vi "efficiency_test.vi"() -> ()   [LabVIEW 2020, in "efficiency_test.lvlib"]
uses:
  efficiency_test.lvlib
  typedefs/test_inputs.ctl
  typedefs/test_results.ctl
  typedefs/instrument_resources.ctl
  <vilib>/addons/_JKI Toolkits/State Machine/_JKI_lib_State_Machine.llb/Select State(s)_err__jki_lib_state_machine.vi
  drivers/Agilent 34401/Public/Data/Read (Single Point).vi
  drivers/Agilent 34401/Agilent 34401.lvlib
  drivers/Agilent 33XXX Series/Agilent 33XXX Series.lvlib
  drivers/Agilent E364X Series/Agilent E364X Series.lvlib
  drivers/Agilent B2900 Series/Agilent B2900 Series.lvlib
panel:
  in  "UI Tab":enum32{"Test", "Instrument Resources"}(tab)
  out "Efficiency (%) vs ILoad (A)":T1(graph) caption="XY Graph - dark"
  in  "test_inputs":T2={"Vin (V)"=36.0, "Iin Limit (A)"=0.1, "ILoad Start (A)"=0.0, "ILoad Stop (A)"=10.0, "ILoad Step (A)"=1.0, "Vdd (V)"=36.0, "IVdd Limit (A)"=0.1} {"IVdd Limit (A)" format="%#_6p"; "Vdd (V)" format="%#_6p"; "ILoad Step (A)" format="%#_6p"; "ILoad Stop (A)" format="%#_6p"; "ILoad Start (A)" format="%#_6p"; "Iin Limit (A)" format="%#_6p"; "Vin (V)" format="%#_6p"}
  out "Output Results":T3
  in  "instrument_resources":T4={"Vin Voltage DMM"="Vin_Volt", "Vin Current DMM"="Vin_Current", "Vout Voltage DMM"="Vout Voltage DMM", "Vout Current DMM"="Vout_Current", "Eload"="Eload", "FSW_Source"="FSW", "Vin_supply"="Vin_supply", "Vdd_supply"="Vin_supply"}
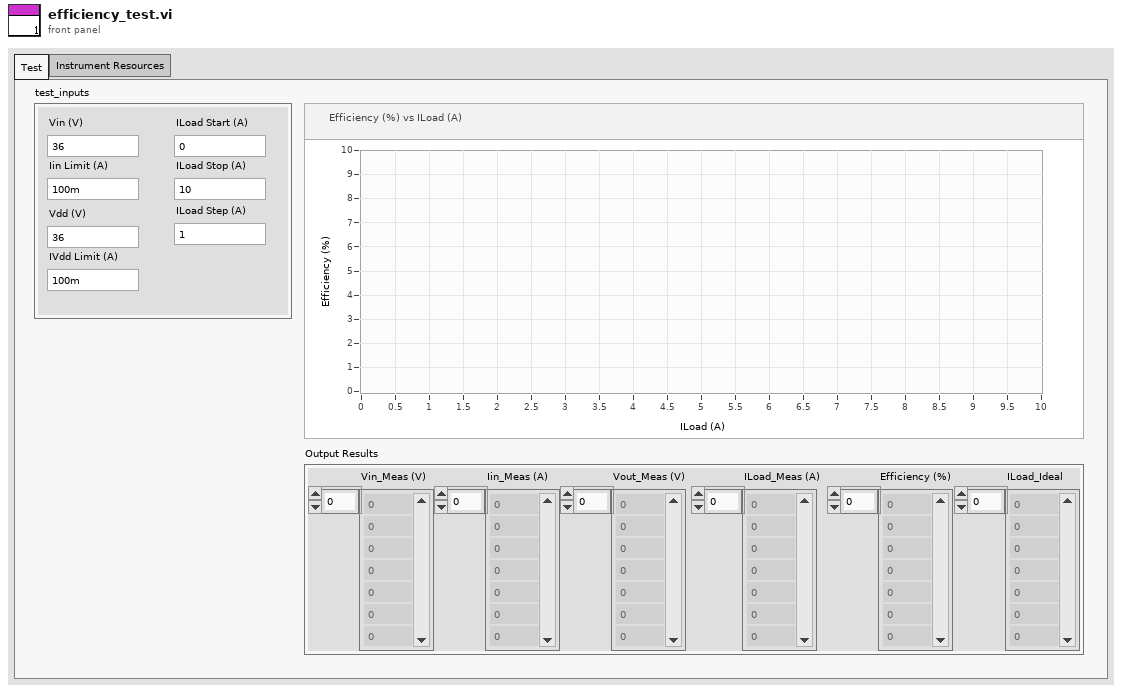
[diagram p1: front panel]
types:
  T1 = cluster{"ILoad (A)":dbl[], "Efficiency (%) ":dbl[]}
  T2 = typedef "efficiency_test.lvlib/test_inputs.ctl" = cluster{"Vin (V)":dbl, "Iin Limit (A)":dbl, "ILoad Start (A)":dbl, "ILoad Stop (A)":dbl, "ILoad Step (A)":dbl, "Vdd (V)":dbl, "IVdd Limit (A)":dbl}
  T3 = typedef "efficiency_test.lvlib/test_results.ctl" = cluster{"Vin_Meas (V)":dbl[], "Iin_Meas (A)":dbl[], "Vout_Meas (V)":dbl[], "ILoad_Meas (A)":dbl[], "Efficiency (%)":dbl[], "ILoad_Ideal":dbl[]}
  T4 = typedef "efficiency_test.lvlib/instrument_resources.ctl" = cluster{"Vin Voltage DMM":refnum<visa-resource-name>, "Vin Current DMM":refnum<visa-resource-name>, "Vout Voltage DMM":refnum<visa-resource-name>, "Vout Current DMM":refnum<visa-resource-name>, "Eload":refnum<visa-resource-name>, "FSW_Source":refnum<visa-resource-name>, "Vin_supply":refnum<visa-resource-name>, "Vdd_supply":refnum<visa-resource-name>}
  T5 = cluster{"test_inputs":T2, "output_results":T3, "instrument_resources":T4, "ILoad Sweep Current":dbl[]}
  T6 = cluster{"ILoad_Meas (A)":dbl[], "Efficiency (%)":dbl[]}
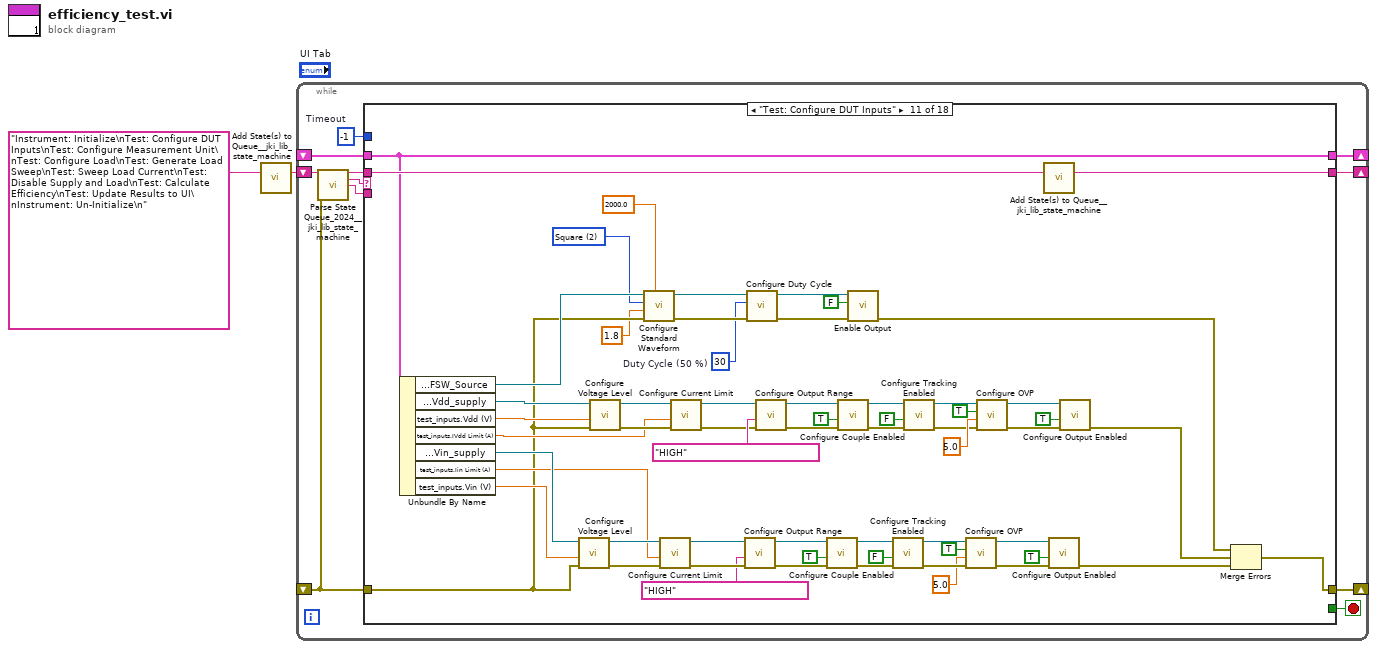
[diagram p0: block diagram]
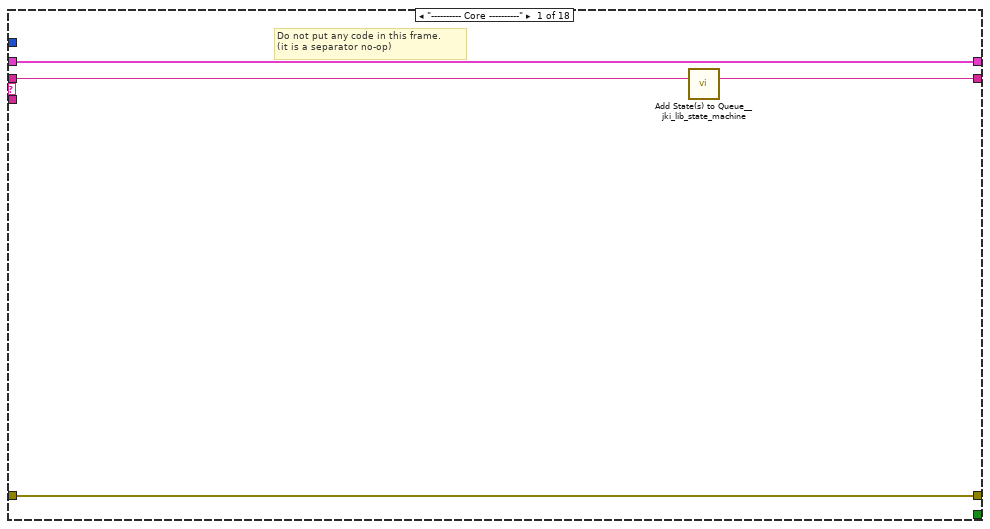
[diagram p2: hidden frame]
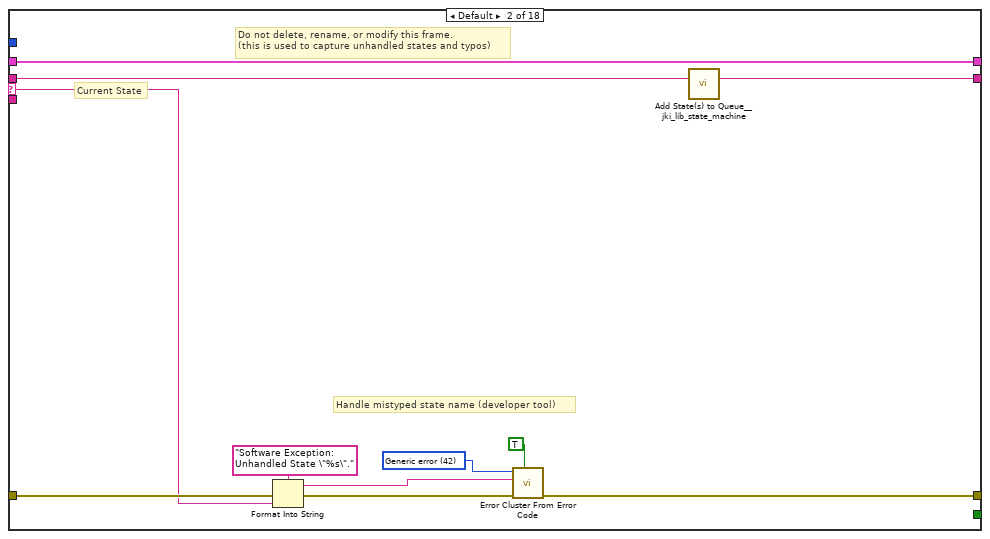
[diagram p3: hidden frame]
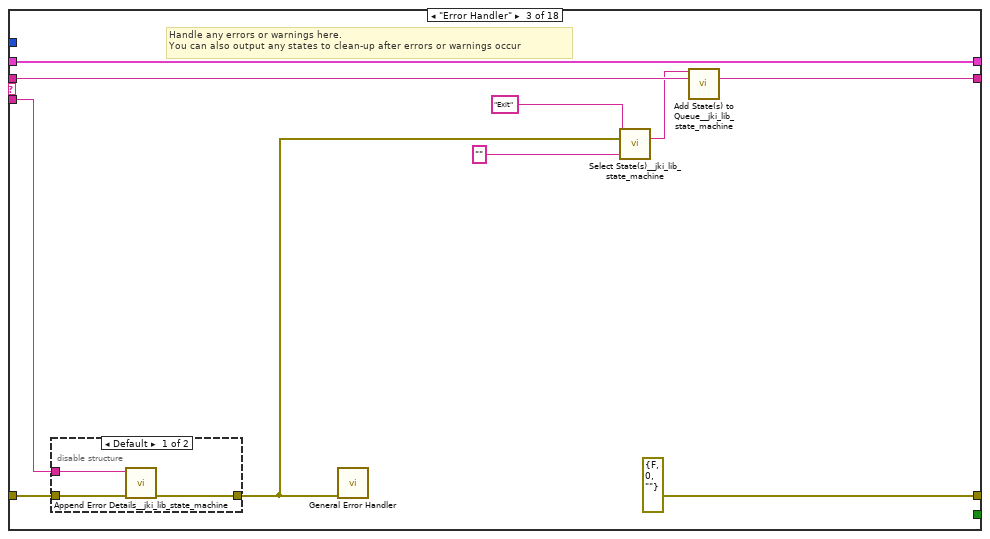
[diagram p4: hidden frame]
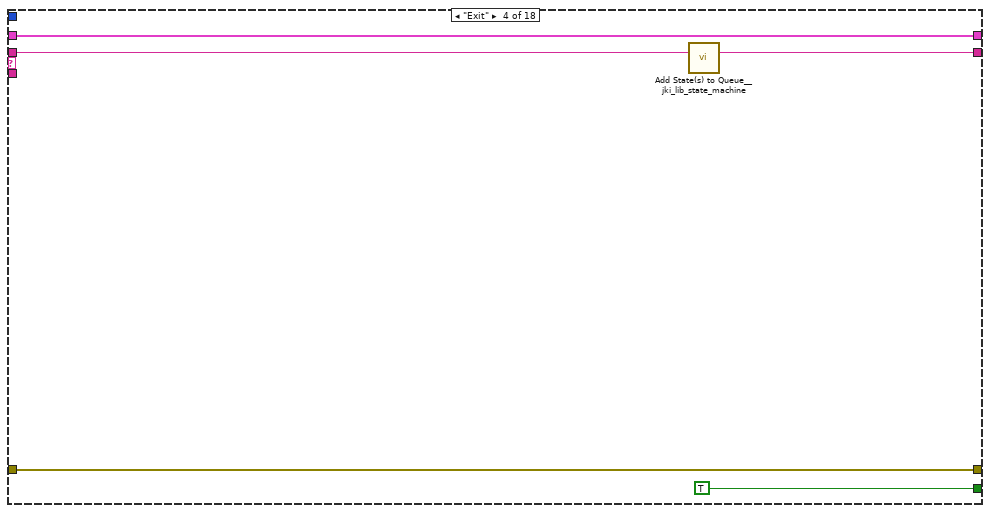
[diagram p6: hidden frame]
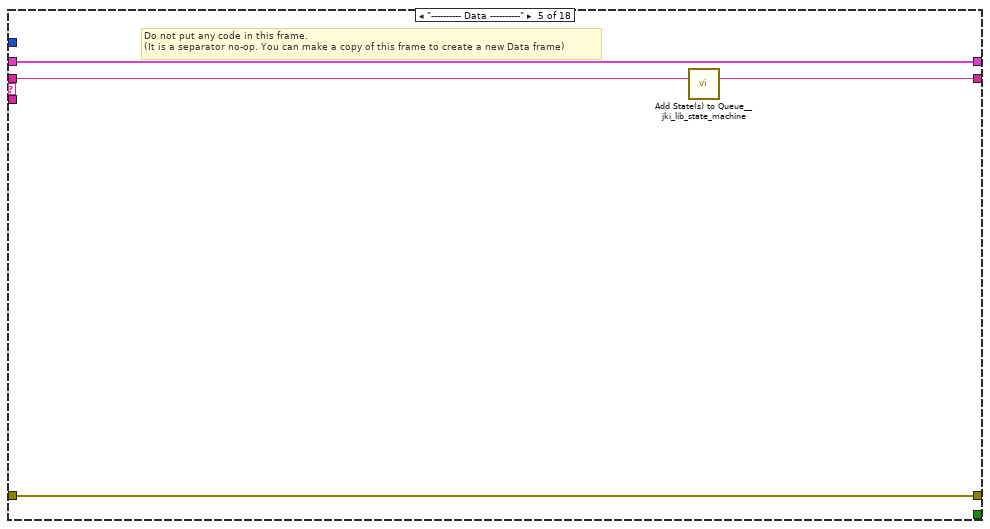
[diagram p7: hidden frame]
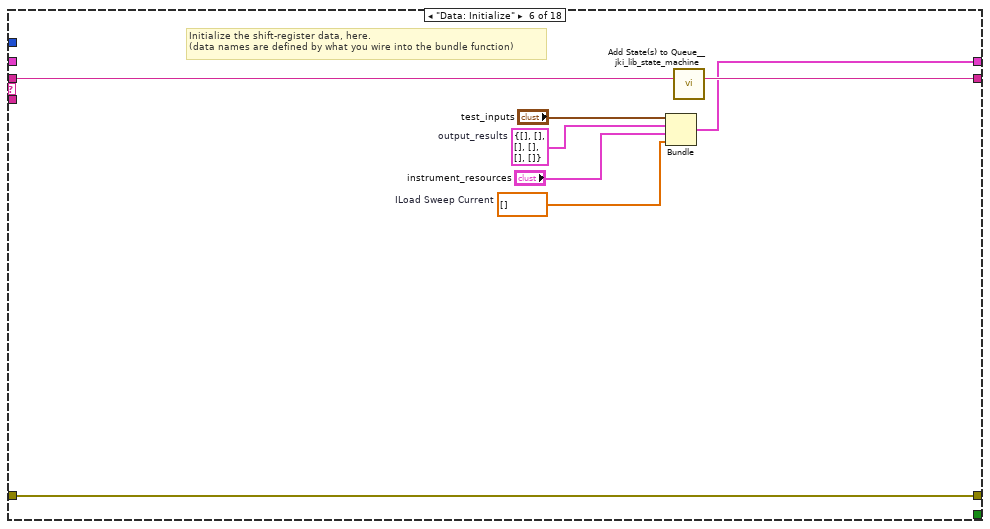
[diagram p8: hidden frame]
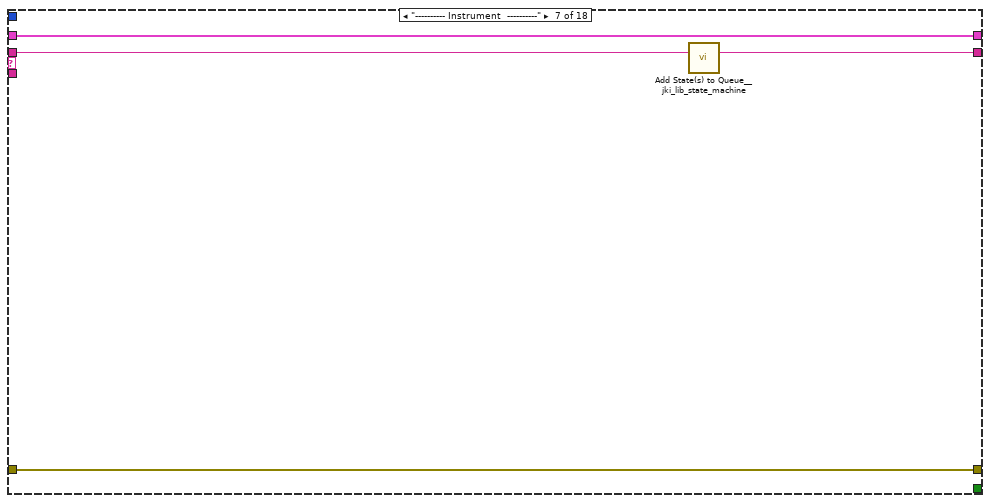
[diagram p9: hidden frame]
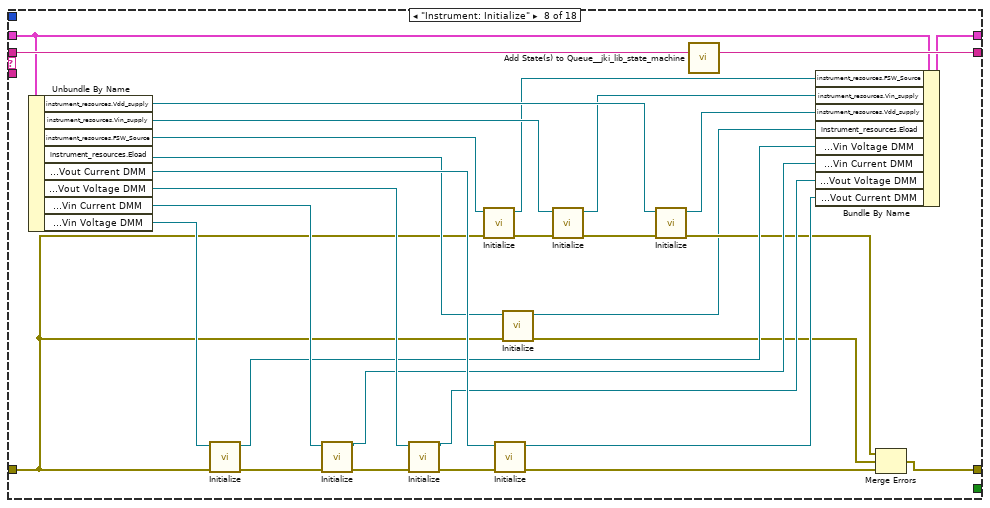
[diagram p10: hidden frame]
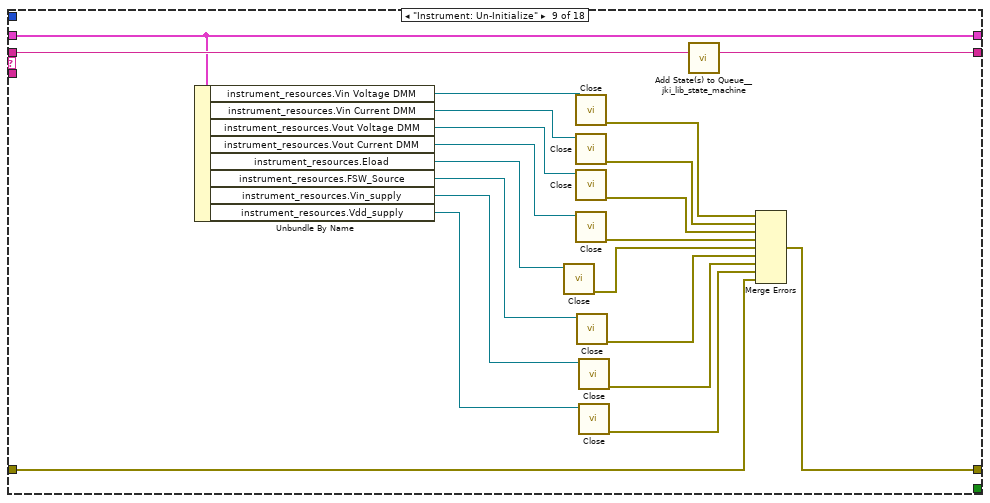
[diagram p11: hidden frame]
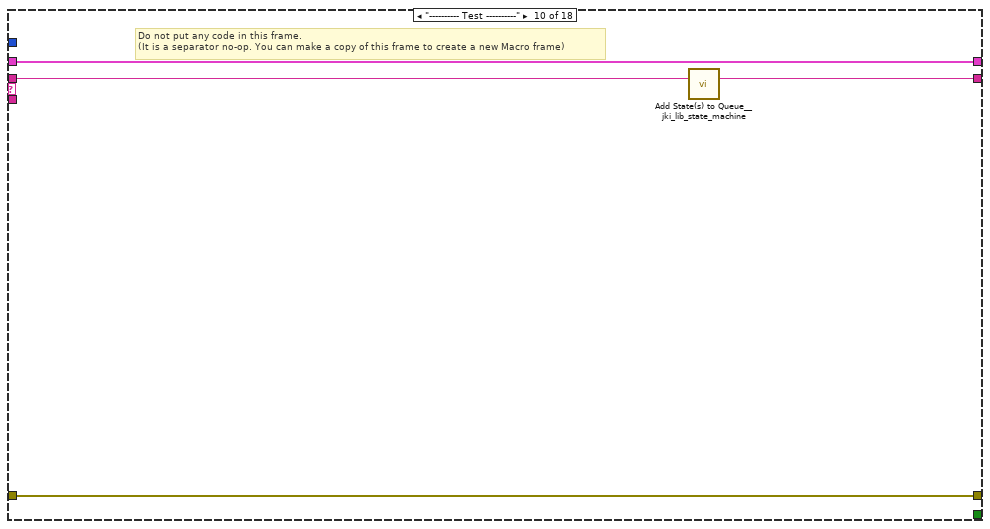
[diagram p12: hidden frame]
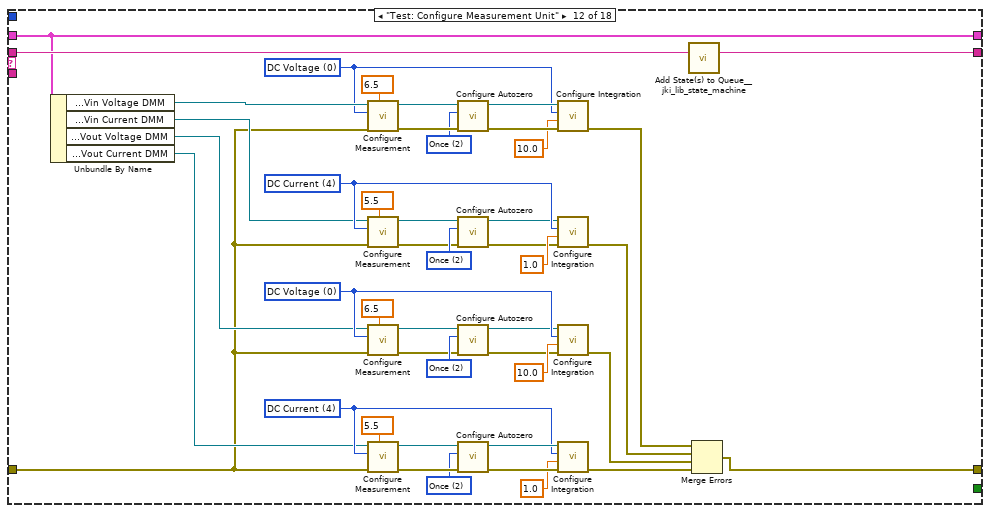
[diagram p13: hidden frame]
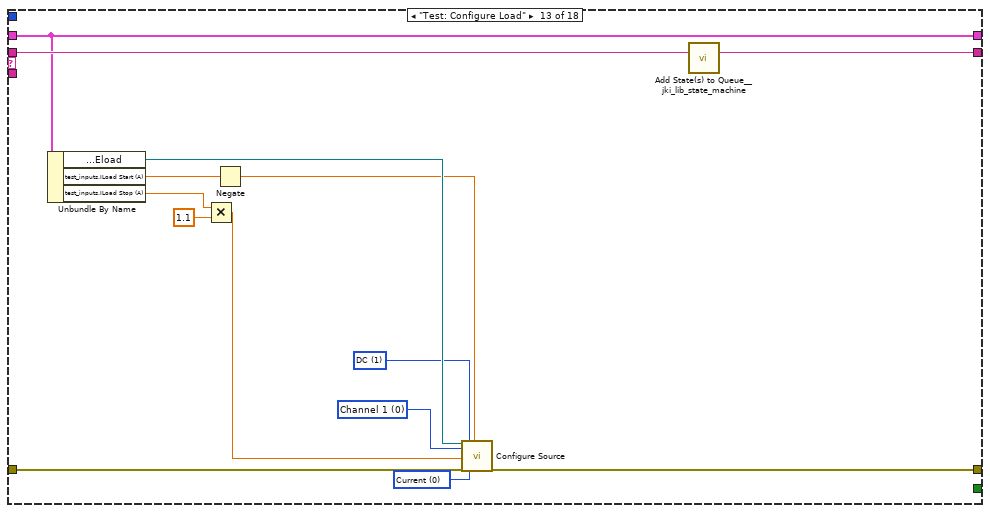
[diagram p14: hidden frame]
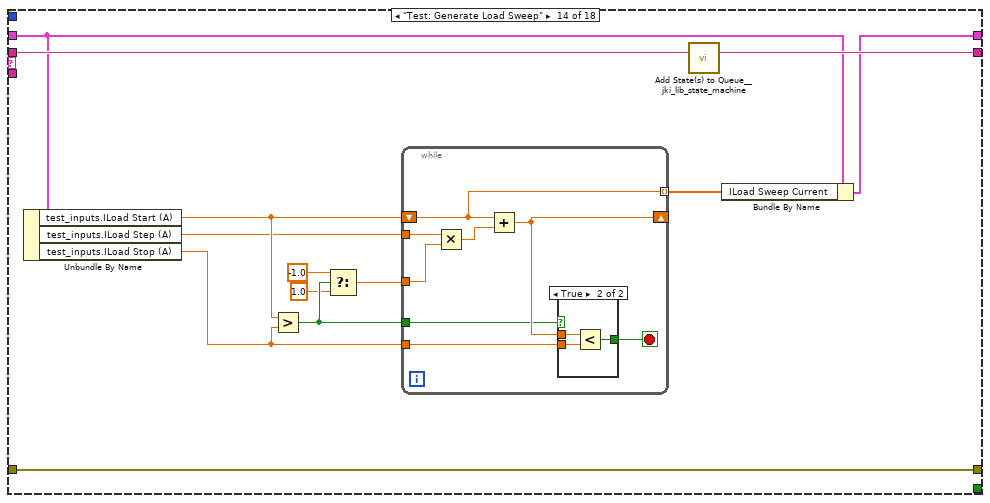
[diagram p15: hidden frame]
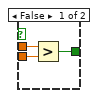
[diagram p16: hidden frame]
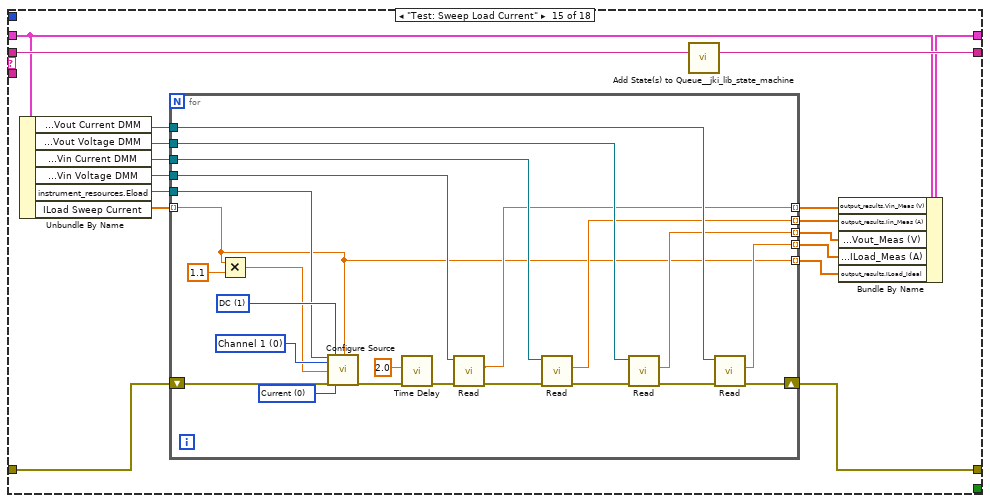
[diagram p17: hidden frame]
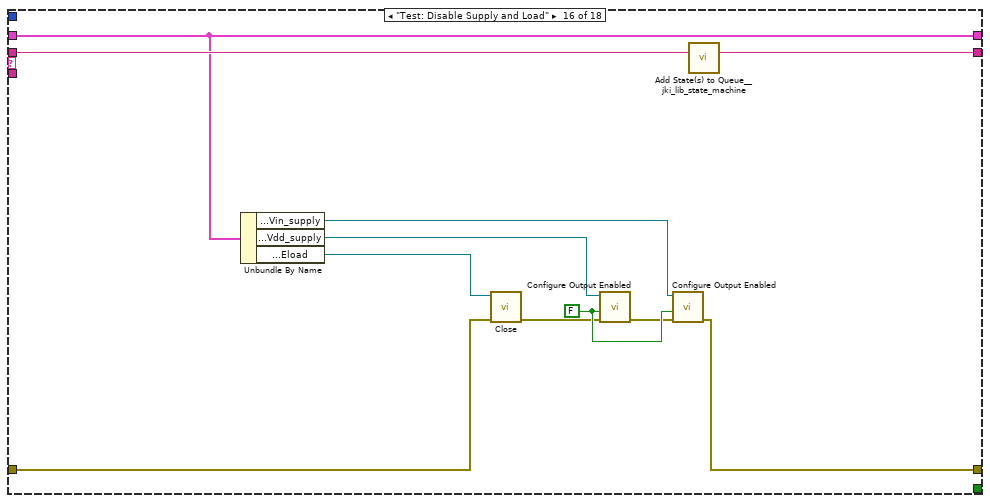
[diagram p18: hidden frame]
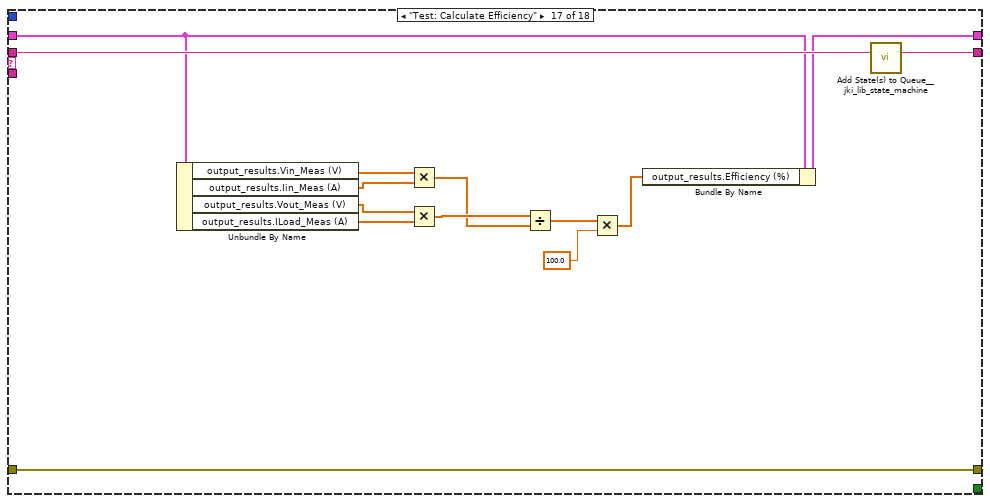
[diagram p19: hidden frame]
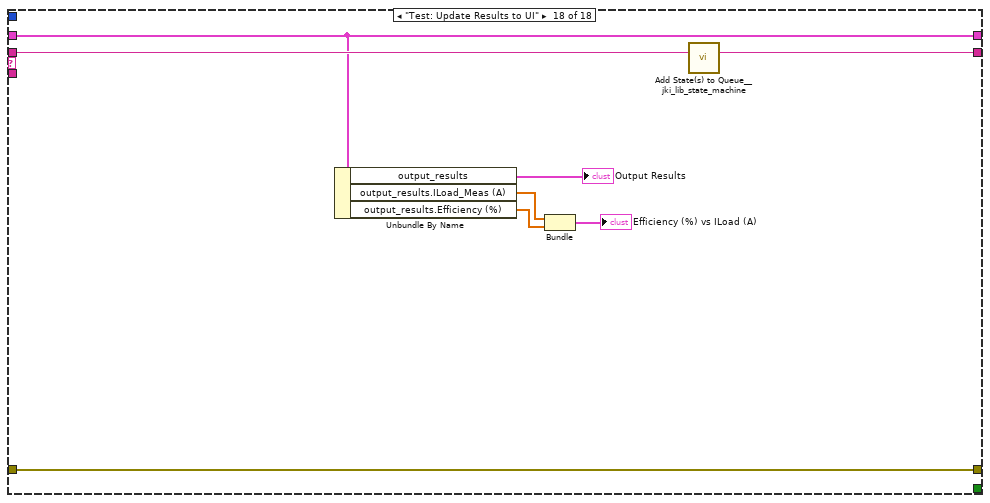
[diagram p20: hidden frame]
diagram:
  n1 = call <vilib>:"Add State(s) to Queue__jki_lib_state_machine.vi"("State(s) in (\"\")"="Instrument: Initialize\nTest: Configure DUT Inputs\nTest: Configure Measurement Unit\nTest: Configure Load\nTest: Generate Load Sweep\nTest: Sweep Load Current\nTest: Disable Supply and Load\nTest: Calculate Efficiency\nTest: Update Results to UI\nInstrument: Un-Initialize\n") -> ("States Out"=w2:string)  [unwired: 14 in]
  n2 = while {
    shift-right: [w6] -> _
    shift-left: _ -> [w5]
    shift-right: [w9] -> _
    shift-left: _ -> [w3]
    shift-right: [w8] -> _
    shift-left: w2 -> [w10]
    stop <- w7 stop-if-true
    w4 = -1  # Timeout
    n3 = call <vilib>:"Parse State Queue_2024__jki_lib_state_machine.vi"("State Queue"=w10, "Error In (no error)"=w3) -> ("Remaining States"=w12:string, "Current State"=w13:string, "Arguments"=w11:string)  [unwired: 11 in]
    n4 = case shown="\"Test: Configure DUT Inputs\"" w13 {
      selector: w13 -> [_ w18 _ _ _ _ _ _ _ _ _ _ _ _ _ _ _ _]
      tunnel: w12 -> [w17 w22 w38 w47 w51 w59 w63 w93 w114 w118 w178 w223 w237 w250 w281 w315 w329 w337]
      tunnel: w11 -> [_ _ w33 _ _ _ _ _ _ _ _ _ _ _ _ _ _ _]
      tunnel: w5 -> [w14 w20 w35 w45 w48 _ w60 w71 w112 w115 w176 w221 w235 w238 w267 w313 w316 w334]
      tunnel: [w15 w24 errorcluster {"status"=FALSE, "code"=0, "source"=""} ("error out") w44 w49 w56 w61 w68 w97 w116 w119 w179 w230 w248 w266 w308 w327 w335] -> w9
      tunnel: w3 -> [w15 w23 w34 w44 w49 w56 w61 w65 w96 w116 w132 w184 w231 w248 w265 w306 w327 w335]
      tunnel: [w16 w21 w37 w46 w50 w58 w62 w92 w113 w117 w177 w222 w236 w249 w280 w314 w328 w336] -> w8
      tunnel: [_ _ _ TRUE _ _ _ _ _ _ _ _ _ _ _ _ _ _] -> w7
      tunnel: [w14 w20 w35 w45 w48 w57 w60 w72 w112 w115 w176 w221 w235 w239 w268 w313 w317 w334] -> w6
      tunnel: w4 -> [_ _ _ _ _ _ _ _ _ _ _ _ _ _ _ _ _ _]
      frame "---------- Core ----------" {
        # "Do not put any code in this frame.\n(it is a separator no-op)"
        n5 = call <vilib>:"Add State(s) to Queue__jki_lib_state_machine.vi"("State(s) in (\"\")"=w17) -> ("States Out"=w16:string)  [unwired: 14 in]
      }
      frame Default {
        w27 = 42 items=["No error", "Argument error", "Memory is full", "Out of zone", "End of file", "File already open", "Generic file I/O error", "File not found", "File permission error", "Disk is full", "Duplicate path", "Too many files open", "System feature not enabled", "Resource file not found", "Cannot add resource", "Resource not found", "Image not found", "Image memory error", "Pen does not exist", "Config type invalid", "Config token not found", "Config parse error", "Config memory error", "Bad external code format", "Bad external code offset", "External code not present", "Null window", "Destroy window error", "Null menu", "Print aborted", "Bad print record", "Print driver error", "Windows error during printing", "Memory error during printing", "Print dialog error", "Generic print error", "Invalid device refnum", "Device not found", "Device parameter error", "Device unit error", "Cannot open device", "Device call aborted", "Generic error", "Cancelled by user", "Object ID too low", "Object ID too high", "Object not in heap", "Unknown heap", "Unknown object (invalid DefProc)", "Unknown object (DefProc not in table)", "Message out of range", "Invalid (null) method", "Unknown message", "Manager call not supported", "Bad address", "Network operation in progress", "Network operation timed out", "Connection is busy", "Network attribute not supported", "Network error", "Address in use", "System out of memory", "Connection aborted", "Connection refused", "Not connected", "Already connected", "Connection closed", "Initialization error (interapplication manager)", "Bad occurrence", "Wait on unbound occurrence handler", "Occurrence queue overflow", "Datalog type conflict", "Unused", "Unrecognized type (interapplication manager)", "Memory corrupt", "Failed to make temporary DLL", "Old CIN version", "Drag socket not found", "Failed to load drop-object", "Failed to register OLE object", "Failed to release OLE object", "Format specifier type mismatch", "Unknown format specifier", "Too few format specifiers", "Too many format specifiers", "Scan failed", "Newer CIN version", "Error converting to variant", "Runtime menu error", "Password tampered", "Variant attribute not found", "Incompatible variant data type", "Event data is not available", "Event Store is not present", "Occurrence is not found", "Event Queue is not created", "Event info is not available", "Refnum passed is NULL", "Error retrieving Class GUID", "Error retrieving CoClass GUID", "Error retrieving TypeLib GUID.", "Bad built application magic bytes.", "Specific driver is different from the specific driver associated with the Logical Name.", "There is no session opened to the class driver.", "Max Error", "MAX - Error with config objects", "MAX - Error loading configuration", "MAX - Group not supported"]
        # "Current State"
        # "Do not delete, rename, or modify this frame.\n(this is used to capture unhandled states and typos)"
        # "Handle mistyped state name (developer tool)"
        n6 = Format Into String(format string="Software Exception: Unhandled State \"%s\"." ("message"), error in=w23, w18) -> (resulting string=w26:string, error out=w25:errorcluster)  [unwired: 1 in]
        n7 = call <vilib>:"Error Cluster From Error Code.vi"("show call chain? (False)"=TRUE, "error in (no error)"=w25, "error message (\"\")"=w26, "error code (0)"=w27) -> ("error out"=w24:errorcluster)  [unwired: 5 in]
        n8 = call <vilib>:"Add State(s) to Queue__jki_lib_state_machine.vi"("State(s) in (\"\")"=w22) -> ("States Out"=w21:string)  [unwired: 14 in]
      }
      frame "Error Handler" {
        # "Handle any errors or warnings here.\nYou can also output any states to clean-up after errors or warnings occur"
        n9 = disable-structure shown="Default" {
          disable-tunnel: w34 -> [w41 w42]
          disable-tunnel: w33 -> [w40 _]
          disable-tunnel: [w39 w42] -> w32
          frame condition #0 (active) {
            n10 = call <vilib>:"Append Error Details__jki_lib_state_machine.vi"("error in (no error)"=w41, "Previous State and Argument(s)"=w40) -> ("error out"=w39:errorcluster)  [unwired: 9 in]
          }
          frame condition #1 {
          }
        }
        n11 = call <vilib>:"General Error Handler.vi"("error in (no error)"=w32) -> ()  [unwired: 10 in, 5 out]
        n12 = call-poly <vilib>:"Select State(s)__jki_lib_state_machine.vi"("State(s) if True (\"\")"="Exit", "Select"=w32, "State(s) if False (\"\")"="") -> ("States Out"=w30:string)  [unwired: 12 in]
        n13 = call <vilib>:"Add State(s) to Queue__jki_lib_state_machine.vi"("State(s) in Front (\"\")"=w30, "State(s) in (\"\")"=w38) -> ("States Out"=w37:string)  [unwired: 13 in]
      }
      frame "Exit" {
        n14 = call <vilib>:"Add State(s) to Queue__jki_lib_state_machine.vi"("State(s) in (\"\")"=w47) -> ("States Out"=w46:string)  [unwired: 14 in]
      }
      frame "---------- Data ----------" {
        # "Do not put any code in this frame.\n(It is a separator no-op. You can make a copy of this frame to create a new Data frame)"
        n15 = call <vilib>:"Add State(s) to Queue__jki_lib_state_machine.vi"("State(s) in (\"\")"=w51) -> ("States Out"=w50:string)  [unwired: 14 in]
      }
      frame "Data: Initialize" {
        w52 = dbl[] []  # ILoad Sweep Current
        w54 = T3 {"Vin_Meas (V)"=[], "Iin_Meas (A)"=[], "Vout_Meas (V)"=[], "ILoad_Meas (A)"=[], "Efficiency (%)"=[], "ILoad_Ideal"=[]}  # output_results
        # "Initialize the shift-register data, here.\n(data names are defined by what you wire into the bundle function)"
        n16 = Bundle("test_inputs"="test_inputs", "output_results"=w54, "instrument_resources"="instrument_resources", "ILoad Sweep Current"=w52) -> (w57:T5)  [unwired: 1 in]
        n17 = call <vilib>:"Add State(s) to Queue__jki_lib_state_machine.vi"("State(s) in (\"\")"=w59) -> ("States Out"=w58:string)  [unwired: 14 in]
      }
      frame "---------- Instrument  ----------" {
        n18 = call <vilib>:"Add State(s) to Queue__jki_lib_state_machine.vi"("State(s) in (\"\")"=w63) -> ("States Out"=w62:string)  [unwired: 14 in]
      }
      frame "Instrument: Initialize" {
        n19 = Unbundle By Name(w71) -> ("instrument_resources.Vdd_supply"=w84:refnum<visa-resource-name>, "instrument_resources.Vin_supply"=w85:refnum<visa-resource-name>, "instrument_resources.FSW_Source"=w86:refnum<visa-resource-name>, "instrument_resources.Eload"=w67:refnum<visa-resource-name>, "instrument_resources.Vout Current DMM"=w80:refnum<visa-resource-name>, "instrument_resources.Vout Voltage DMM"=w81:refnum<visa-resource-name>, "instrument_resources.Vin Current DMM"=w82:refnum<visa-resource-name>, "instrument_resources.Vin Voltage DMM"=w83:refnum<visa-resource-name>)
        n20 = call "Initialize.vi"("error in (no error)"=w65, "VISA resource name"=w83) -> ("error out"=w89:errorcluster, "VISA resource name out"=w76:refnum<visa-resource-name>)  [unwired: 8 in]
        n21 = call "Initialize.vi"("error in (no error)"=w89, "VISA resource name"=w82) -> ("error out"=w91:errorcluster, "VISA resource name out"=w75:refnum<visa-resource-name>)  [unwired: 8 in]
        n22 = call "Initialize.vi"("error in (no error)"=w91, "VISA resource name"=w81) -> ("error out"=w90:errorcluster, "VISA resource name out"=w74:refnum<visa-resource-name>)  [unwired: 8 in]
        n23 = call "Initialize.vi"("error in (no error)"=w65, "VISA resource name"=w86) -> ("error out"=w88:errorcluster, "VISA resource name out"=w79:refnum<visa-resource-name>)  [unwired: 8 in]
        n24 = call "Initialize.vi"("error in (no error)"=w90, "VISA resource name"=w80) -> ("error out"=w69:errorcluster, "VISA resource name out"=w73:refnum<visa-resource-name>)  [unwired: 8 in]
        n25 = call "Initialize.vi"("error in (no error)"=w65, "VISA resource name"=w67) -> ("error out"=w64:errorcluster, "VISA resource name out"=w66:refnum<visa-resource-name>)  [unwired: 8 in]
        n26 = call "Initialize.vi"("error in (no error)"=w88, "VISA resource name"=w85) -> ("error out"=w87:errorcluster, "VISA resource name out"=w78:refnum<visa-resource-name>)  [unwired: 8 in]
        n27 = call "Initialize.vi"("error in (no error)"=w87, "VISA resource name"=w84) -> ("error out"=w70:errorcluster, "VISA resource name out"=w77:refnum<visa-resource-name>)  [unwired: 8 in]
        n28 = call <vilib>:"Add State(s) to Queue__jki_lib_state_machine.vi"("State(s) in (\"\")"=w93) -> ("States Out"=w92:string)  [unwired: 14 in]
        n29 = Bundle By Name(cluster=w71, "instrument_resources.FSW_Source"=w79, "instrument_resources.Vin_supply"=w78, "instrument_resources.Vdd_supply"=w77, "instrument_resources.Eload"=w66, "instrument_resources.Vin Voltage DMM"=w76, "instrument_resources.Vin Current DMM"=w75, "instrument_resources.Vout Voltage DMM"=w74, "instrument_resources.Vout Current DMM"=w73) -> (w72:T5)
        n30 = Merge Errors(w70, w64, w69) -> (w68:errorcluster)
      }
      frame "Instrument: Un-Initialize" {
        n31 = Unbundle By Name(w112) -> ("instrument_resources.Vin Voltage DMM"=w111:refnum<visa-resource-name>, "instrument_resources.Vin Current DMM"=w110:refnum<visa-resource-name>, "instrument_resources.Vout Voltage DMM"=w109:refnum<visa-resource-name>, "instrument_resources.Vout Current DMM"=w108:refnum<visa-resource-name>, "instrument_resources.Eload"=w95:refnum<visa-resource-name>, "instrument_resources.FSW_Source"=w107:refnum<visa-resource-name>, "instrument_resources.Vin_supply"=w106:refnum<visa-resource-name>, "instrument_resources.Vdd_supply"=w105:refnum<visa-resource-name>)
        n32 = call "Close.vi"("VISA resource name"=w95) -> ("error out"=w94:errorcluster)  [unwired: 10 in]
        n33 = call "Close.vi"("VISA resource name"=w111) -> ("error out"=w104:errorcluster)  [unwired: 10 in]
        n34 = call "Close.vi"("VISA resource name"=w110) -> ("error out"=w103:errorcluster)  [unwired: 10 in]
        n35 = call "Close.vi"("VISA resource name"=w109) -> ("error out"=w102:errorcluster)  [unwired: 10 in]
        n36 = call "Close.vi"("VISA resource name"=w108) -> ("error out"=w101:errorcluster)  [unwired: 10 in]
        n37 = call "Close.vi"("VISA resource name"=w107) -> ("error out"=w100:errorcluster)  [unwired: 10 in]
        n38 = call "Close.vi"("VISA resource name"=w106) -> ("error out"=w99:errorcluster)  [unwired: 10 in]
        n39 = call "Close.vi"("VISA resource name"=w105) -> ("error out"=w98:errorcluster)  [unwired: 10 in]
        n40 = call <vilib>:"Add State(s) to Queue__jki_lib_state_machine.vi"("State(s) in (\"\")"=w114) -> ("States Out"=w113:string)  [unwired: 14 in]
        n41 = Merge Errors(w104, w103, w102, w101, w94, w100, w99, w98, w96) -> (w97:errorcluster)
      }
      frame "---------- Test ----------" {
        # "Do not put any code in this frame.\n(It is a separator no-op. You can make a copy of this frame to create a new Macro frame)"
        n42 = call <vilib>:"Add State(s) to Queue__jki_lib_state_machine.vi"("State(s) in (\"\")"=w118) -> ("States Out"=w117:string)  [unwired: 14 in]
      }
      frame "Test: Configure DUT Inputs" {
        w124 = 30  # Duty Cycle (50 %)
        w127 = u16 2 items=["DC", "Sine", "Square", "Triangle", "Ramp", "Pulse", "Noise", "Sinc", "Negative Ramp", "Exponential Rise", "Exponential Fall", "Cardiac"] ("Waveform Function (1: Sine)")
        n43 = Unbundle By Name(w176) -> ("instrument_resources.FSW_Source"=w133:refnum<visa-resource-name>, "instrument_resources.Vdd_supply"=w136:refnum<visa-resource-name>, "test_inputs.Vdd (V)"=w135:dbl, "test_inputs.IVdd Limit (A)"=w134:dbl, "instrument_resources.Vin_supply"=w175:refnum<visa-resource-name>, "test_inputs.Iin Limit (A)"=w155:dbl, "test_inputs.Vin (V)"=w156:dbl)
        n44 = call "Configure Voltage Level.vi"("error in (no error)"=w132, "Level (0.0 Volts)"=w156, "VISA resource name"=w175) -> ("error out"=w174:errorcluster, "VISA resource name out"=w170:refnum<visa-resource-name>)  [unwired: 7 in]
        n45 = call "Configure Voltage Level.vi"("error in (no error)"=w132, "Level (0.0 Volts)"=w135, "VISA resource name"=w136) -> ("error out"=w137:errorcluster, "VISA resource name out"=w141:refnum<visa-resource-name>)  [unwired: 7 in]
        n46 = call "Configure Standard Waveform.vi"("Frequency (1000 Hz)"=2000.0, "error in (no error)"=w132, "Amplitude (1)"=1.8, "Waveform Function (1: Sine)"=w127, "VISA resource name"=w133) -> ("error out"=w131:errorcluster, "VISA resource name out"=w129:refnum<visa-resource-name>)  [unwired: 5 in]
        n47 = call "Configure Current Limit.vi"("error in (no error)"=w174, "Current Limit (0.0 Amps)"=w155, "VISA resource name"=w170) -> ("error out"=w173:errorcluster, "VISA resource name out"=w169:refnum<visa-resource-name>)  [unwired: 7 in]
        n48 = call "Configure Current Limit.vi"("error in (no error)"=w137, "Current Limit (0.0 Amps)"=w134, "VISA resource name"=w141) -> ("error out"=w138:errorcluster, "VISA resource name out"=w142:refnum<visa-resource-name>)  [unwired: 7 in]
        n49 = call "Configure Output Range.vi"("error in (no error)"=w173, "Range (High Voltage / Low Current)"="HIGH", "VISA resource name"=w169) -> ("error out"=w172:errorcluster, "VISA resource name out"=w168:refnum<visa-resource-name>)  [unwired: 7 in]
        n50 = call "Configure Duty Cycle.vi"("error in (no error)"=w131, "Duty Cycle (50 %)"=w124, "VISA resource name"=w129) -> ("error out"=w130:errorcluster, "VISA resource name out"=w128:refnum<visa-resource-name>)  [unwired: 7 in]
        n51 = call "Configure Output Range.vi"("error in (no error)"=w138, "Range (High Voltage / Low Current)"="HIGH", "VISA resource name"=w142) -> ("error out"=w139:errorcluster, "VISA resource name out"=w143:refnum<visa-resource-name>)  [unwired: 7 in]
        n52 = call "Configure Couple Enabled.vi"("error in (no error)"=w172, "Coupling Enabled (F: Off)"=TRUE, "VISA resource name"=w168) -> ("error out"=w171:errorcluster, "VISA resource name out"=w167:refnum<visa-resource-name>)  [unwired: 7 in]
        n53 = call "Configure Couple Enabled.vi"("error in (no error)"=w139, "Coupling Enabled (F: Off)"=TRUE, "VISA resource name"=w143) -> ("error out"=w140:errorcluster, "VISA resource name out"=w144:refnum<visa-resource-name>)  [unwired: 7 in]
        n54 = call "Enable Output.vi"("error in (no error)"=w130, "Enable Output  (T: Enable)"=FALSE, "VISA resource name"=w128) -> ("error out"=w120:errorcluster)  [unwired: 7 in, 1 out]
        n55 = call "Configure Tracking Enabled.vi"("error in (no error)"=w171, "Tracking Enabled (F: Off)"=FALSE, "VISA resource name"=w167) -> ("error out"=w163:errorcluster, "VISA resource name out"=w161:refnum<visa-resource-name>)  [unwired: 7 in]
        n56 = call "Configure Tracking Enabled.vi"("error in (no error)"=w140, "Tracking Enabled (F: Off)"=FALSE, "VISA resource name"=w144) -> ("error out"=w148:errorcluster, "VISA resource name out"=w150:refnum<visa-resource-name>)  [unwired: 7 in]
        n57 = call "Configure OVP.vi"("error in (no error)"=w163, "Limit (22.0 Volts)"=5.0, "OVP Enabled (T: On)"=TRUE, "VISA resource name"=w161) -> ("error out"=w159:errorcluster, "VISA resource name out"=w158:refnum<visa-resource-name>)  [unwired: 6 in]
        n58 = call "Configure OVP.vi"("error in (no error)"=w148, "Limit (22.0 Volts)"=5.0, "OVP Enabled (T: On)"=TRUE, "VISA resource name"=w150) -> ("error out"=w152:errorcluster, "VISA resource name out"=w153:refnum<visa-resource-name>)  [unwired: 6 in]
        n59 = call <vilib>:"Add State(s) to Queue__jki_lib_state_machine.vi"("State(s) in (\"\")"=w178) -> ("States Out"=w177:string)  [unwired: 14 in]
        n60 = call "Configure Output Enabled.vi"("error in (no error)"=w159, "Output Enabled (F: Off)"=TRUE, "VISA resource name"=w158) -> ("error out"=w122:errorcluster)  [unwired: 7 in, 1 out]
        n61 = call "Configure Output Enabled.vi"("error in (no error)"=w152, "Output Enabled (F: Off)"=TRUE, "VISA resource name"=w153) -> ("error out"=w121:errorcluster)  [unwired: 7 in, 1 out]
        n62 = Merge Errors(w120, w121, w122) -> (w119:errorcluster)
      }
      frame "Test: Configure Measurement Unit" {
        w195 = 5.5 items=["4.5"=4.5, "5.5"=5.5, "6.5"=6.5] ("Manual Resolution (5.5 Digits)")
        w196 = u16 2 items=["On", "Off", "Once"] ("Autozero  (0: On)")
        w197 = 1.0 items=["0.001"=0.001, "0.002"=0.002, "0.006"=0.006, "0.02"=0.02, "0.06"=0.06, "0.2"=0.2, "1"=1.0, "10"=10.0, "100"=100.0] ("Integration Time (1 PLCs)")
        w198 = u16 4 items=["DC Voltage", "AC Voltage", "2 - Wire Resistance", "4 - Wire Resistance", "DC Current", "AC Current", "Frequency", "Period", "Continuity", "Diode Checking", "VDC:VDC Ratio", "Temperature", "Capacitance"] ("Function (0: DC Voltage)")
        w194 = 6.5 items=["4.5"=4.5, "5.5"=5.5, "6.5"=6.5] ("Manual Resolution (5.5 Digits)")
        w193 = u16 2 items=["On", "Off", "Once"] ("Autozero  (0: On)")
        w192 = 10.0 items=["0.001"=0.001, "0.002"=0.002, "0.006"=0.006, "0.02"=0.02, "0.06"=0.06, "0.2"=0.2, "1"=1.0, "10"=10.0, "100"=100.0] ("Integration Time (1 PLCs)")
        w191 = u16 0 items=["DC Voltage", "AC Voltage", "2 - Wire Resistance", "4 - Wire Resistance", "DC Current", "AC Current", "Frequency", "Period", "Continuity", "Diode Checking", "VDC:VDC Ratio", "Temperature", "Capacitance"] ("Function (0: DC Voltage)")
        w211 = 5.5 items=["4.5"=4.5, "5.5"=5.5, "6.5"=6.5] ("Manual Resolution (5.5 Digits)")
        w210 = u16 2 items=["On", "Off", "Once"] ("Autozero  (0: On)")
        w209 = 1.0 items=["0.001"=0.001, "0.002"=0.002, "0.006"=0.006, "0.02"=0.02, "0.06"=0.06, "0.2"=0.2, "1"=1.0, "10"=10.0, "100"=100.0] ("Integration Time (1 PLCs)")
        w208 = u16 4 items=["DC Voltage", "AC Voltage", "2 - Wire Resistance", "4 - Wire Resistance", "DC Current", "AC Current", "Frequency", "Period", "Continuity", "Diode Checking", "VDC:VDC Ratio", "Temperature", "Capacitance"] ("Function (0: DC Voltage)")
        w212 = 6.5 items=["4.5"=4.5, "5.5"=5.5, "6.5"=6.5] ("Manual Resolution (5.5 Digits)")
        w213 = u16 2 items=["On", "Off", "Once"] ("Autozero  (0: On)")
        w214 = 10.0 items=["0.001"=0.001, "0.002"=0.002, "0.006"=0.006, "0.02"=0.02, "0.06"=0.06, "0.2"=0.2, "1"=1.0, "10"=10.0, "100"=100.0] ("Integration Time (1 PLCs)")
        w215 = u16 0 items=["DC Voltage", "AC Voltage", "2 - Wire Resistance", "4 - Wire Resistance", "DC Current", "AC Current", "Frequency", "Period", "Continuity", "Diode Checking", "VDC:VDC Ratio", "Temperature", "Capacitance"] ("Function (0: DC Voltage)")
        n63 = Unbundle By Name(w221) -> ("instrument_resources.Vin Voltage DMM"=w220:refnum<visa-resource-name>, "instrument_resources.Vin Current DMM"=w203:refnum<visa-resource-name>, "instrument_resources.Vout Voltage DMM"=w186:refnum<visa-resource-name>, "instrument_resources.Vout Current DMM"=w185:refnum<visa-resource-name>)
        n64 = call "Configure Measurement.vi"("Manual Resolution (5.5 Digits)"=w212, "error in (no error)"=w184, "Function (0: DC Voltage)"=w215, "VISA resource name"=w220) -> ("error out"=w218:errorcluster, "VISA resource name out"=w219:refnum<visa-resource-name>)  [unwired: 6 in]
        n65 = call "Configure Measurement.vi"("Manual Resolution (5.5 Digits)"=w211, "error in (no error)"=w184, "Function (0: DC Voltage)"=w208, "VISA resource name"=w203) -> ("error out"=w205:errorcluster, "VISA resource name out"=w204:refnum<visa-resource-name>)  [unwired: 6 in]
        n66 = call "Configure Measurement.vi"("Manual Resolution (5.5 Digits)"=w194, "error in (no error)"=w184, "Function (0: DC Voltage)"=w191, "VISA resource name"=w186) -> ("error out"=w188:errorcluster, "VISA resource name out"=w187:refnum<visa-resource-name>)  [unwired: 6 in]
        n67 = call "Configure Measurement.vi"("Manual Resolution (5.5 Digits)"=w195, "error in (no error)"=w184, "Function (0: DC Voltage)"=w198, "VISA resource name"=w185) -> ("error out"=w201:errorcluster, "VISA resource name out"=w202:refnum<visa-resource-name>)  [unwired: 6 in]
        n68 = call "Configure Autozero.vi"("error in (no error)"=w218, "Autozero  (0: On)"=w213, "VISA resource name"=w219) -> ("error out"=w217:errorcluster, "VISA resource name out"=w216:refnum<visa-resource-name>)  [unwired: 7 in]
        n69 = call "Configure Autozero.vi"("error in (no error)"=w205, "Autozero  (0: On)"=w210, "VISA resource name"=w204) -> ("error out"=w206:errorcluster, "VISA resource name out"=w207:refnum<visa-resource-name>)  [unwired: 7 in]
        n70 = call "Configure Autozero.vi"("error in (no error)"=w188, "Autozero  (0: On)"=w193, "VISA resource name"=w187) -> ("error out"=w189:errorcluster, "VISA resource name out"=w190:refnum<visa-resource-name>)  [unwired: 7 in]
        n71 = call "Configure Autozero.vi"("error in (no error)"=w201, "Autozero  (0: On)"=w196, "VISA resource name"=w202) -> ("error out"=w200:errorcluster, "VISA resource name out"=w199:refnum<visa-resource-name>)  [unwired: 7 in]
        n72 = call "Configure Integration.vi"("error in (no error)"=w217, "Integration Time (1 PLCs)"=w214, "Function (0: DC Voltage)"=w215, "VISA resource name"=w216) -> ("error out"=w180:errorcluster)  [unwired: 6 in, 1 out]
        n73 = call "Configure Integration.vi"("error in (no error)"=w206, "Integration Time (1 PLCs)"=w209, "Function (0: DC Voltage)"=w208, "VISA resource name"=w207) -> ("error out"=w181:errorcluster)  [unwired: 6 in, 1 out]
        n74 = call "Configure Integration.vi"("error in (no error)"=w189, "Integration Time (1 PLCs)"=w192, "Function (0: DC Voltage)"=w191, "VISA resource name"=w190) -> ("error out"=w182:errorcluster)  [unwired: 6 in, 1 out]
        n75 = call "Configure Integration.vi"("error in (no error)"=w200, "Integration Time (1 PLCs)"=w197, "Function (0: DC Voltage)"=w198, "VISA resource name"=w199) -> ("error out"=w183:errorcluster)  [unwired: 6 in, 1 out]
        n76 = call <vilib>:"Add State(s) to Queue__jki_lib_state_machine.vi"("State(s) in (\"\")"=w223) -> ("States Out"=w222:string)  [unwired: 14 in]
        n77 = Merge Errors(w180, w181, w182, w183) -> (w179:errorcluster)
      }
      frame "Test: Configure Load" {
        w224 = 0 items=["Current", "Voltage"] ("Source Mode (1: Voltage)")
        w225 = 1 items=["Pulse", "DC"] ("Source Shape (1: DC)")
        w228 = 0 items=["Channel 1", "Channel 2"] ("Channel (0: Channel 1)")
        n78 = Unbundle By Name(w235) -> ("instrument_resources.Eload"=w229:refnum<visa-resource-name>, "test_inputs.ILoad Start (A)"=w234:dbl, "test_inputs.ILoad Stop (A)"=w232:dbl)
        n79 = Multiply(x=w232, y=1.1) -> (x*y=w227:dbl)
        n80 = Negate(x=w234) -> (-x=w226:dbl)
        n81 = call "Configure Source.vi"("VISA resource name"=w229, "Channel (0: Channel 1)"=w228, "Source Range (2)"=w227, "error in (no error)"=w231, "Source Shape (1: DC)"=w225, "Source Mode (1: Voltage)"=w224, "Output Level (0)"=w226) -> ("error out"=w230:errorcluster)  [unwired: 11 in, 1 out]
        n82 = call <vilib>:"Add State(s) to Queue__jki_lib_state_machine.vi"("State(s) in (\"\")"=w237) -> ("States Out"=w236:string)  [unwired: 14 in]
      }
      frame "Test: Generate Load Sweep" {
        n83 = Unbundle By Name(w238) -> ("test_inputs.ILoad Start (A)"=w243:dbl, "test_inputs.ILoad Step (A)"=w242:dbl, "test_inputs.ILoad Stop (A)"=w241:dbl)
        n84 = Greater?(x=w243, y=w241) -> (0:w247:bool)
        n85 = Select(t=-1.0 ("y"), s=w247, f=1.0 ("y")) -> (s? t:f=w244:dbl)
        n86 = while {
          tunnel: w242 -> [w258]
          shift-right: [w256] -> _
          shift-left: w243 -> [w257]
          tunnel: [w257] -> w240 mode=indexing
          tunnel: w241 -> [w255]
          tunnel: w247 -> [w251]
          tunnel: w244 -> [w252]
          stop <- w254 stop-if-true
          n87 = Multiply(x=w258, y=w252) -> (x*y=w253:dbl)
          n88 = Add(x=w257, y=w253) -> (x+y=w256:dbl)
          n89 = case shown="True" w251 {
            tunnel: w256 -> [w260 w264]
            tunnel: w255 -> [w261 w263]
            tunnel: [w259 w262] -> w254
            frame False {
              n90 = Greater?(x=w260, y=w261) -> (0:w259:bool)
            }
            frame True {
              n91 = Less?(x=w264, y=w263) -> (x < y?=w262:bool)
            }
          }
        }
        n92 = call <vilib>:"Add State(s) to Queue__jki_lib_state_machine.vi"("State(s) in (\"\")"=w250) -> ("States Out"=w249:string)  [unwired: 14 in]
        n93 = Bundle By Name(cluster=w238, "ILoad Sweep Current"=w240) -> (w239:T5)
      }
      frame "Test: Sweep Load Current" {
        n94 = Unbundle By Name(w267) -> ("instrument_resources.Vout Current DMM"=w274:refnum<visa-resource-name>, "instrument_resources.Vout Voltage DMM"=w275:refnum<visa-resource-name>, "instrument_resources.Vin Current DMM"=w276:refnum<visa-resource-name>, "instrument_resources.Vin Voltage DMM"=w277:refnum<visa-resource-name>, "instrument_resources.Eload"=w279:refnum<visa-resource-name>, "ILoad Sweep Current"=w278:dbl[])
        n95 = for {
          shift-right: [w302] -> w266
          shift-left: w265 -> [w287]
          tunnel: w279 -> [w285]
          tunnel: w278 -> [w283] mode=indexing
          tunnel: w277 -> [w298]
          tunnel: w276 -> [w297]
          tunnel: w275 -> [w296]
          tunnel: w274 -> [w295]
          tunnel: [w294] -> w273 mode=indexing
          tunnel: [w293] -> w272 mode=indexing
          tunnel: [w292] -> w271 mode=indexing
          tunnel: [w291] -> w270 mode=indexing
          tunnel: [w283] -> w269 mode=indexing
          w288 = 0 items=["Current", "Voltage"] ("Source Mode (1: Voltage)")
          w289 = 1 items=["Pulse", "DC"] ("Source Shape (1: DC)")
          w290 = 0 items=["Channel 1", "Channel 2"] ("Channel (0: Channel 1)")
          n96 = Multiply(x=w283, y=1.1) -> (x*y=w282:dbl)
          n97 = call "Configure Source.vi"("VISA resource name"=w285, "Channel (0: Channel 1)"=w290, "Source Range (2)"=w282, "error in (no error)"=w287, "Source Shape (1: DC)"=w289, "Source Mode (1: Voltage)"=w288, "Output Level (0)"=w283) -> ("error out"=w286:errorcluster)  [unwired: 11 in, 1 out]
          n98 = call "Time Delay"("error in (no error)"=w286, "Delay Time (s)"=2.0) -> ("error out"=w303:errorcluster)  [unwired: 9 in]
          n99 = call-poly "Read.vi"("error in (no error)"=w303, "VISA resource name"=w298) -> ("error out"=w301:errorcluster, "Measurement"=w294:dbl)  [unwired: 7 in, 1 out]
          n100 = call-poly "Read.vi"("error in (no error)"=w301, "VISA resource name"=w297) -> ("error out"=w300:errorcluster, "Measurement"=w293:dbl)  [unwired: 7 in, 1 out]
          n101 = call-poly "Read.vi"("error in (no error)"=w300, "VISA resource name"=w296) -> ("error out"=w299:errorcluster, "Measurement"=w292:dbl)  [unwired: 7 in, 1 out]
          n102 = call-poly "Read.vi"("error in (no error)"=w299, "VISA resource name"=w295) -> ("error out"=w302:errorcluster, "Measurement"=w291:dbl)  [unwired: 7 in, 1 out]
        }
        n103 = call <vilib>:"Add State(s) to Queue__jki_lib_state_machine.vi"("State(s) in (\"\")"=w281) -> ("States Out"=w280:string)  [unwired: 14 in]
        n104 = Bundle By Name(cluster=w267, "output_results.Vin_Meas (V)"=w273, "output_results.Iin_Meas (A)"=w272, "output_results.Vout_Meas (V)"=w271, "output_results.ILoad_Meas (A)"=w270, "output_results.ILoad_Ideal"=w269) -> (w268:T5)
      }
      frame "Test: Disable Supply and Load" {
        w310 = FALSE ("Output Enabled (F: Off)")
        n105 = Unbundle By Name(w313) -> ("instrument_resources.Vin_supply"=w311:refnum<visa-resource-name>, "instrument_resources.Vdd_supply"=w312:refnum<visa-resource-name>, "instrument_resources.Eload"=w305:refnum<visa-resource-name>)
        n106 = call "Close.vi"("error in (no error)"=w306, "VISA resource name"=w305) -> ("error out"=w307:errorcluster)  [unwired: 9 in]
        n107 = call "Configure Output Enabled.vi"("error in (no error)"=w307, "Output Enabled (F: Off)"=w310, "VISA resource name"=w312) -> ("error out"=w309:errorcluster)  [unwired: 7 in, 1 out]
        n108 = call "Configure Output Enabled.vi"("error in (no error)"=w309, "Output Enabled (F: Off)"=w310, "VISA resource name"=w311) -> ("error out"=w308:errorcluster)  [unwired: 7 in, 1 out]
        n109 = call <vilib>:"Add State(s) to Queue__jki_lib_state_machine.vi"("State(s) in (\"\")"=w315) -> ("States Out"=w314:string)  [unwired: 14 in]
      }
      frame "Test: Calculate Efficiency" {
        n110 = Unbundle By Name(w316) -> ("output_results.Vin_Meas (V)"=w326:dbl[], "output_results.Iin_Meas (A)"=w325:dbl[], "output_results.Vout_Meas (V)"=w324:dbl[], "output_results.ILoad_Meas (A)"=w323:dbl[])
        n111 = Multiply(x=w326, y=w325) -> (x*y=w321:dbl[])
        n112 = Multiply(x=w324, y=w323) -> (x*y=w322:dbl[])
        n113 = Divide(x=w322, y=w321) -> (x/y=w320:dbl[])
        n114 = Multiply(x=w320, y=100.0) -> (x*y=w318:dbl[])
        n115 = Bundle By Name(cluster=w316, "output_results.Efficiency (%)"=w318) -> (w317:T5)
        n116 = call <vilib>:"Add State(s) to Queue__jki_lib_state_machine.vi"("State(s) in (\"\")"=w329) -> ("States Out"=w328:string)  [unwired: 14 in]
      }
      frame "Test: Update Results to UI" {
        n117 = Unbundle By Name(w334) -> ("output_results"=→"Output Results":T3, "output_results.ILoad_Meas (A)"=w332:dbl[], "output_results.Efficiency (%)"=w331:dbl[])
        n118 = Bundle("ILoad_Meas (A)"=w332, "Efficiency (%)"=w331) -> (→"Efficiency (%) vs ILoad (A)":T6)  [unwired: 1 in]
        n119 = call <vilib>:"Add State(s) to Queue__jki_lib_state_machine.vi"("State(s) in (\"\")"=w337) -> ("States Out"=w336:string)  [unwired: 14 in]
      }
    }
  }
